vi "Measurement Logic.vi"() -> ()   [LabVIEW 2023, in "GetSineSignal.lvlib"]
uses:
  GetSineSignal.lvlib
  Measurement Configuration.ctl
  Measurement Results.ctl
  <vilib>/MeasurementLink/MeasurementLink Measurement Server/Classes/MeasurementContext/MeasurementContext.lvclass
  <vilib>/Analysis/NI_AALBase.lvlib
panel:
  out "Measurement Context out":refnum<class "MeasurementContext.lvclass">
  in  "Measurement Context":refnum<class "MeasurementContext.lvclass">
  out "Measurement Results":T1
  in  "Measurement Configuration":T2
  out "error out":errorcluster
  in  "error in":errorcluster
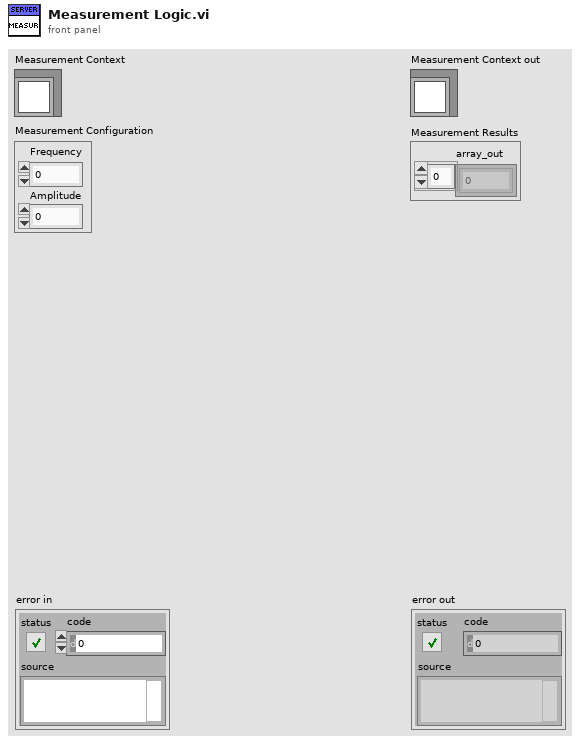
[diagram p1: front panel]
types:
  T1 = typedef "GetSineSignal.lvlib/Measurement Results.ctl" = cluster{"array_out":dbl[]}
  T2 = typedef "GetSineSignal.lvlib/Measurement Configuration.ctl" = cluster{"Frequency":dbl, "Amplitude":dbl}
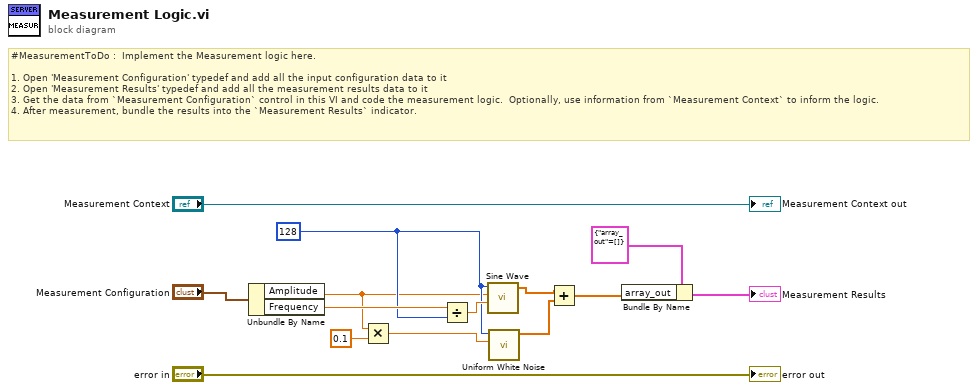
[diagram p0: block diagram]
diagram:
  w7 = 128 ("samples")
  # "#MeasurementToDo :  Implement the Measurement logic here.\n\n1. Open 'Measurement Configuration' typedef and add all the input configuration data to it\n2. Open 'Measurement Results' typedef and add all the measurement results data to it\n3. Get the data from `Measurement Configuration` control in this VI and code the measurement logic.  Optionally, use information from `Measurement Context` to inform the logic.\n4. After measurement, bundle the results into the `Measurement Results` indicator."
  n1 = Unbundle By Name("Measurement Configuration") -> ("Amplitude"=w6:dbl, "Frequency"=w9:dbl)
  n2 = Multiply(x=w6, y=0.1) -> (x*y=w4:dbl)
  n3 = Divide(x=w9, y=w7) -> (x/y=w8:dbl)
  n4 = call <vilib>:"Sine Wave.vi"("samples"=w7, "amplitude"=w6, "frequency"=w8) -> ("sine wave"=w3:dbl[])  [unwired: 2 in, 2 out]
  n5 = call <vilib>:"Uniform White Noise.vi"("amplitude"=w4, "samples"=w7) -> ("uniform white noise"=w2:dbl[])  [unwired: 8 in, 1 out]
  n6 = Add(x=w3, y=w2) -> (x+y=w1:dbl[])
  n7 = Bundle By Name(cluster=T1 {"array_out"=[]} ("Measurement Results"), "array_out"=w1) -> (→"Measurement Results":T1)
  "error out" <- "error in"
  "Measurement Context out" <- "Measurement Context"
